vi "init classes.vi"(8 "error in (no error)":errorcluster, 11 "MVINames":string[](array[string])) -> (0 "error out":errorcluster, 3 "MBs":refnum<class "Master CR.lvclass">[](array[class]))   [LabVIEW 2021, in "Master CR.lvclass"]
uses:
  Master CR.lvclass
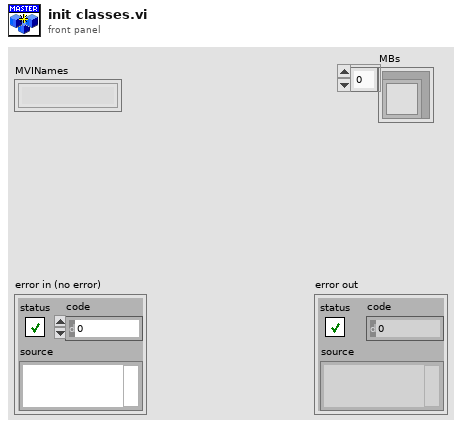
[diagram p1: front panel]
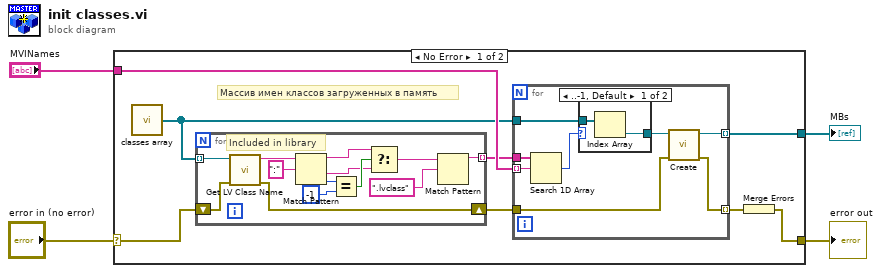
[diagram p0: block diagram]
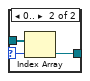
[diagram p2: hidden frame]
diagram:
  n1 = case shown="No Error" "error in (no error)" {
    selector: "error in (no error)" -> [w7 w39]
    tunnel: [w10 w39] -> w3
    tunnel: [w12 _] -> w2
    tunnel: "MVINames" -> [w9 _]
    frame No Error {
      # "Массив имен классов загруженных в память"
      n2 = call "classes array.vi"() -> ("MBs"=w8:refnum<class "Master CR.lvclass">[])
      n3 = for {
        tunnel: w8 -> [w25] mode=indexing
        tunnel: [w22] -> w5 mode=indexing
        shift-right: [w24] -> w6
        shift-left: w7 -> [w21]
        # "Included in library"
        n4 = call <vilib>:"Get LV Class Name.vi"("error in (no error)"=w21, "object"=w25) -> ("error out"=w24:errorcluster, "class name"=w19:string)  [unwired: 8 in]
        n5 = Match Pattern(string=w19, regular expression=":") -> (before substring=w15:string, after substring=w14:string, offset past match=w18:i32)  [unwired: 1 in, 1 out]
        n6 = Equal?(x=w18, y=-1) -> (x = y?=w16:bool)
        n7 = Select(t=w15, s=w16, f=w14) -> (s? t:f=w13:string)
        n8 = Match Pattern(string=w13, regular expression=".lvclass") -> (before substring=w22:string)  [unwired: 1 in, 3 out]
      }
      n9 = for {
        tunnel: [w27] -> w11 mode=indexing
        tunnel: w9 -> [w30] mode=indexing
        tunnel: w8 -> [w33]
        tunnel: w5 -> [w32]
        tunnel: w6 -> [w28]
        tunnel: [w26] -> w12 mode=indexing
        n10 = Search 1D Array(1D array=w32, element=w30) -> (index of element=w31:i32)  [unwired: 1 in]
        n11 = case shown="..-1, Default" w31 {
          selector: w31 -> [_ w36]
          tunnel: w33 -> [w35 w38]
          tunnel: [w34 w37] -> w29
          frame ..-1, Default {
            n12 = Index Array(array=w35) -> (element=w34:refnum<class "Master CR.lvclass">)  [unwired: 1 in]
          }
          frame 0.. {
            n13 = Index Array(array=w38, index=w36) -> (element=w37:refnum<class "Master CR.lvclass">)
          }
        }
        n14 = call-dynamic "Create.vi"("error in (no error)"=w28, "MB in"=w29) -> ("error out"=w27:errorcluster, "MB out"=w26:refnum<class "Master CR.lvclass">)  [unwired: 8 in]
      }
      n15 = Merge Errors(w11) -> (w10:errorcluster)
    }
    frame Error {
    }
  }
  "error out" <- w3
  "MBs" <- w2
